vi "SH_readTrainData.vi"(8 "error in (no error)":errorcluster, 9 "ControlRefs":T1, 10 "NumberOfChannels":i32, 11 "ShapeletClass in":refnum<class "Shapelets Search Brute Force.lvclass">) -> (0 "error out":errorcluster, 3 "ShapeletClass out":refnum<class "Shapelets Search Brute Force.lvclass">)   [LabVIEW 2016, in "Shapelets Search (Brute Force).lvlib" / "Shapelets Search Brute Force.lvclass"]
uses:
  Shapelets Search Brute Force.lvclass
  Shapelets Search Brute Force.lvclass/Shapelets Search Brute Force.ctl
  <vilib>/xml/Load XML File.vi
  <vilib>/xml/Close Reference(Node).vi
  _XML_EEG_Features/XML_EEG_Features.lvlib
  <vilib>/xml/NI_XML.lvlib
panel:
  # "This VI is a part of BCI Design library, http://www.ru-bci.org \nCopyright © 2020, Sotnikov Peter, All rights reserved. License: CC BY-NC 4.0"
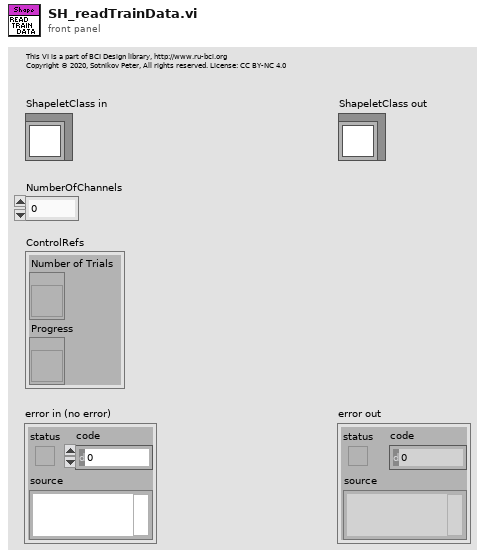
[diagram p1: front panel]
types:
  T1 = cluster{"Number of Trials":refnum<vi>, "Progress":refnum<vi>}
  T2 = typedef "XML_EEG_Features.lvlib/XML_FF_Header.ctl" = cluster{"NumberOfTrials":i32, "NumberOfClasses":i32, "FeatureVectorLength":i32, "FeatureExtractionMethod":string}
  T3 = typedef "XML_EEG_Features.lvlib/XML_FF_Trial.ctl" = cluster{"ClassLabel":string, "FeatureVector":dbl[]}
  T4 = cluster{"ClassLabel":string, "FeatureVector":dbl[][]}
  T5 = cluster{"ClassLabel":string, "FeatureVector":dbl[][]}[]
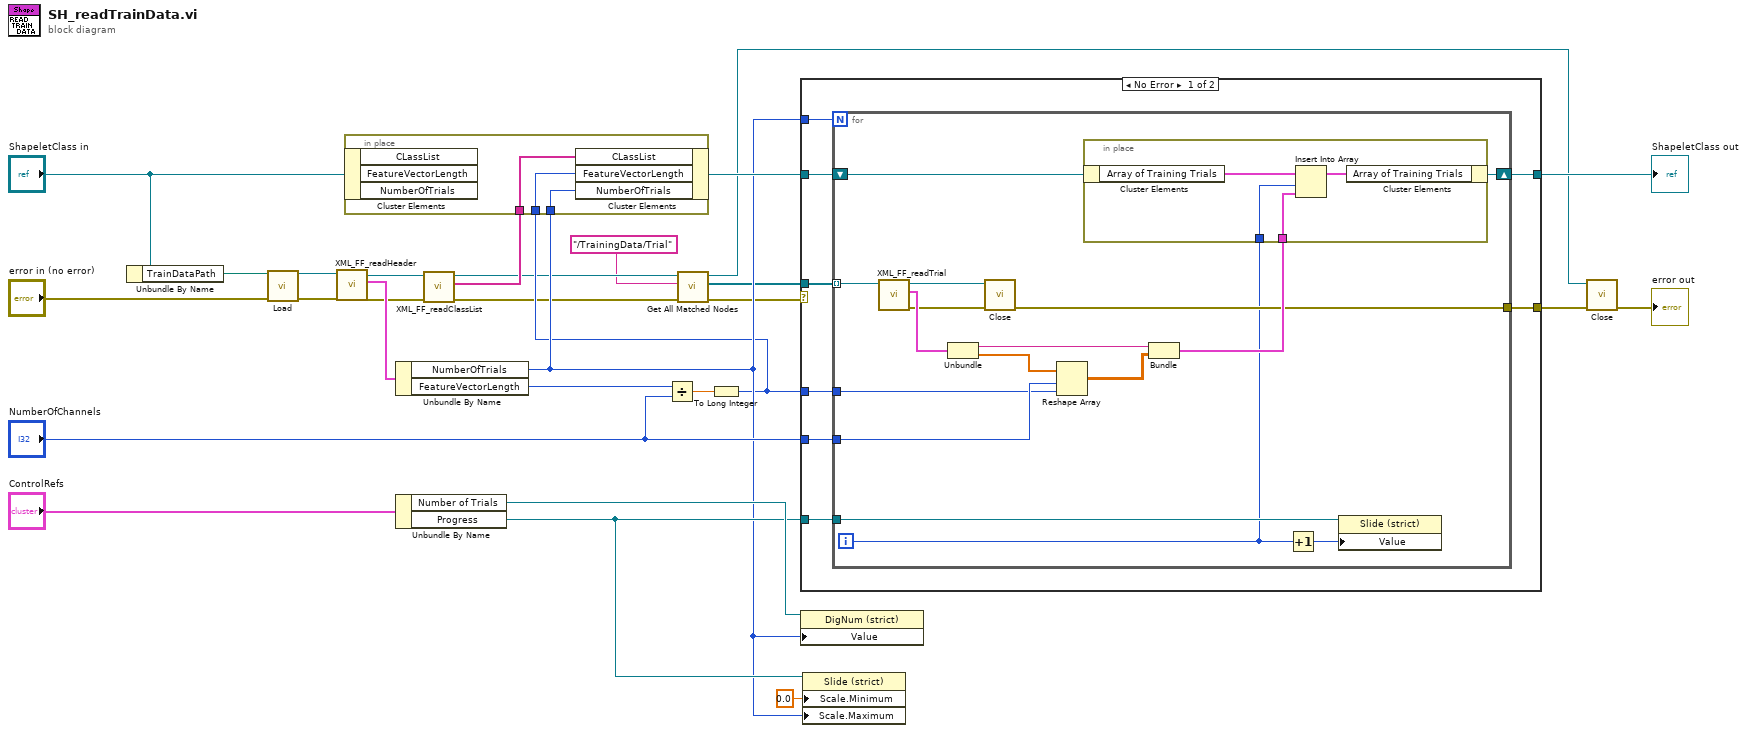
[diagram p0: block diagram]
diagram:
  n1 = Unbundle By Name("ShapeletClass in") -> ("TrainDataPath"=w13:path)
  n2 = call-poly <vilib>:"Load.vi"("path to XML document"=w13, "error in (no error)"="error in (no error)") -> ("DOM document out"=w27:refnum<k20>, "error out"=w28:errorcluster)  [unwired: 11 in, 1 out]
  n3 = call "XML_FF_readHeader.vi"("error in (no error)"=w28, "DOM document in"=w27) -> ("error out"=w17:errorcluster, "FF_Header out"=w26:T2, "DOM document out"=w18:refnum<k20>)  [unwired: 7 in]
  n4 = Unbundle By Name(w26) -> ("NumberOfTrials"=w8:i32, "FeatureVectorLength"=w9:i32)
  n5 = Unbundle By Name("ControlRefs") -> ("Number of Trials"=w21:refnum<vi>, "Progress"=w19:refnum<vi>)
  n6 = call "XML_FF_readClassList.vi"("error in (no error)"=w17, "DOM document in"=w18) -> ("error out"=w6:errorcluster, "CLassLabels out"=w16:string[], "DOM document out"=w5:refnum<k20>)  [unwired: 7 in]
  n7 = Divide(x=w9, y="NumberOfChannels") -> (x/y=w23:dbl)
  n8 = call <vilib>:"Get All Matched Nodes.vi"("error in (no error)"=w6, "XPath expression"="/TrainingData/Trial", "node in"=w5) -> ("error out"=w2:errorcluster, "node result array"=w3:refnum<k20>[], "node out"=w1:refnum<k20>)  [unwired: 6 in]
  n9 = To Long Integer(number=w23) -> (32bit integer=w7:i32)
  n10 = in-place {
    in-place-border: w16 -> [w31]
    in-place-border: w8 -> [w30]
    in-place-border: w7 -> [w29]
    n11 = in-place-cluster #1("ShapeletClass in") -> ()  [unwired: 3 out]
    n12 = in-place-cluster #1("CLassList"=w31, "FeatureVectorLength"=w29, "NumberOfTrials"=w30) -> (w15:refnum<class "Shapelets Search Brute Force.lvclass">)
  }
  n13 = case shown="No Error" w2 {
    selector: w2 -> [_ w60]
    tunnel: w3 -> [w38 _]
    tunnel: w8 -> [w39 _]
    tunnel: w15 -> [w37 w61]
    tunnel: "NumberOfChannels" -> [w33 _]
    tunnel: w7 -> [w32 _]
    tunnel: [w36 w61] -> w11
    tunnel: [w35 w60] -> w24
    tunnel: w19 -> [w34 _]
    frame No Error {
      n14 = for {
        N: w39 -> [_]
        tunnel: w38 -> [w55] mode=indexing
        shift-right: [w53] -> w36
        shift-left: w37 -> [w54]
        tunnel: [w42] -> w35
        tunnel: w34 -> [w52]
        tunnel: w33 -> [w49]
        tunnel: w32 -> [w48]
        i -> [w40]
        n15 = call "XML_FF_readTrial.vi"("DOM document in"=w55) -> ("error out"=w44:errorcluster, "Trial out"=w51:T3, "DOM document out"=w43:refnum<k20>)  [unwired: 8 in]
        n16 = Unbundle(w51) -> ("ClassLabel"=w47:string, "FeatureVector"=w50:dbl[])
        n17 = call-poly <vilib>:"Close.vi"("error in (no error)"=w44, "node"=w43) -> ("error out"=w42:errorcluster)  [unwired: 7 in]
        n18 = Reshape Array(w50, w49, w48) -> (w46:dbl[][])
        n19 = Bundle("ClassLabel"=w47, "FeatureVector"=w46) -> (w45:T4)  [unwired: 1 in]
        n20 = in-place {
          in-place-border: w40 -> [w57]
          in-place-border: w45 -> [w56]
          n21 = in-place-cluster #2(w54) -> ("Array of Training Trials"=w59:T5)
          n22 = Insert Into Array(array=w59, index=w57, new element=w56) -> (w58:T5)
          n23 = in-place-cluster #2("Array of Training Trials"=w58) -> (w53:refnum<class "Shapelets Search Brute Force.lvclass">)
        }
        n24 = Increment(x=w40) -> (x+1=w41:i32)
        n25 = property class="Slide (strict)"(reference=w52, "Value"=w41) -> ()  [unwired: 1 in, 2 out]
      }
    }
    frame Error {
    }
  }
  "ShapeletClass out" <- w11
  n26 = property class="DigNum (strict)"(reference=w21, "Value"=w8) -> ()  [unwired: 1 in, 2 out]
  n27 = property class="Slide (strict)"(reference=w19, "Scale.Minimum"=0.0 ("Data Entry Limits:Minimum"), "Scale.Maximum"=w8) -> ()  [unwired: 1 in, 2 out]
  n28 = call-poly <vilib>:"Close.vi"("error in (no error)"=w24, "node"=w1) -> ("error out"=→"error out":errorcluster)  [unwired: 7 in]
